vi "setHPSubnet.vi"(8 "error in (no error)":errorcluster, 10 "Modbus":refnum<class "IModbus.lvclass">, 11 "ILCCommunications in":refnum<class "ILCCommunications.lvclass">) -> (0 "error out":errorcluster, 3 "ILCCommunications out":refnum<class "ILCCommunications.lvclass">)   [LabVIEW 2016, in "ILCCommunications.lvclass"]
uses:
  ILCCommunications.lvclass
  Common_RT_Modbus/IModbus/IModbus.lvclass
  ILCCommunications.lvclass/ILCCommunications.ctl
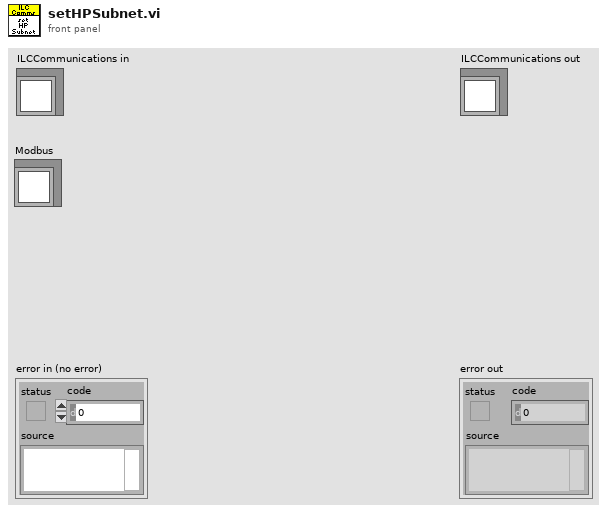
[diagram p1: front panel]
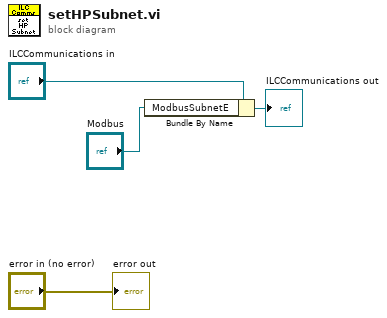
[diagram p0: block diagram]
diagram:
  n1 = Bundle By Name(cluster="ILCCommunications in", "ModbusSubnetE"="Modbus") -> (→"ILCCommunications out":refnum<class "ILCCommunications.lvclass">)
  "error out" <- "error in (no error)"
